vi "Test Remove Nested Test Class from Suite.vi"(8 "error in (no error)":errorcluster, 11 "LUnit Test Suite Tests in":refnum<class "LUnit Test Suite Tests.lvclass">) -> (0 "error out":errorcluster, 3 "LUnit Test Suite Tests out":refnum<class "LUnit Test Suite Tests.lvclass">)   [LabVIEW 2020, in "LUnit Test Suite Tests.lvclass"]
uses:
  LUnit Test Suite Tests.lvclass
  C:/Program Files (x86)/National Instruments/LabVIEW 2020/vi.lib/Astemes/LUnit/Test Case.lvclass
  Test Doubles/Test Case Test Double/Test Case Test Double.lvclass
  <vilib>/Astemes/LUnit/Test Case.lvclass/Test Case.ctl
  <vilib>/Astemes/LUnit/Core/LUnit Test Case/Private/Append Fail Result.vi
  <vilib>/Astemes/LUnit/Core/LUnit Test Case/Private/Append Pass Result.vi
  <vilib>/Astemes/LUnit/Core/LUnit Test Case/Private/Run In UI.vi
  <vilib>/Utility/error.llb/Clear Errors.vi
  source/Core/LUnit Test Suite/LUnit Test Suite.lvclass
  C:/git/astemes-lunit/source/Core/Runnable/Runnable.lvclass
  <vilib>/Astemes/LUnit/Test Case.lvclass
panel:
  out "List of Runnables":string[](array[string])
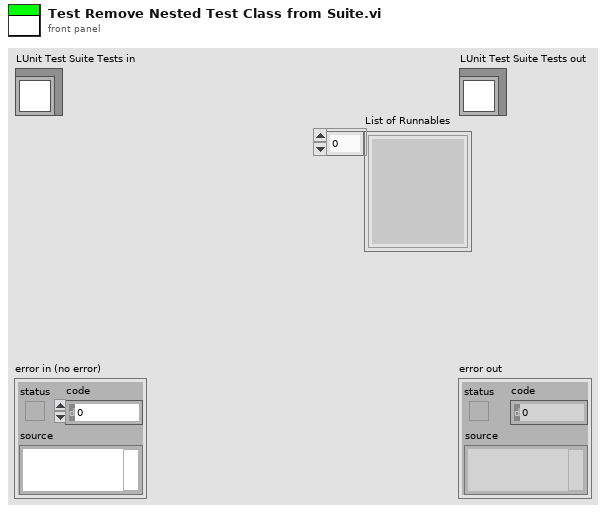
[diagram p1: front panel]
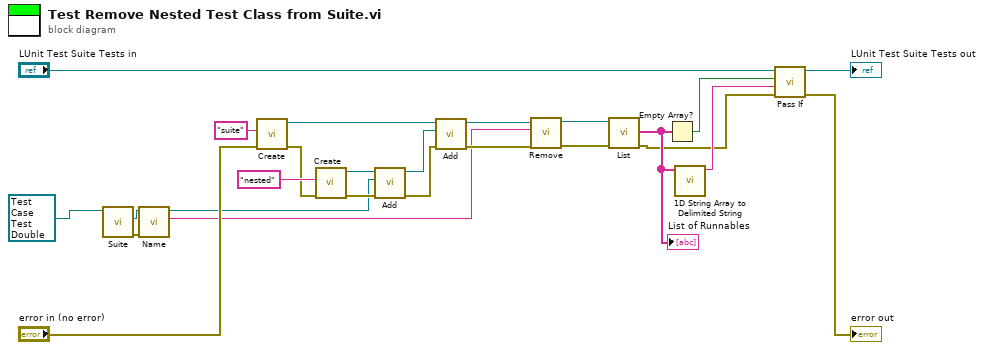
[diagram p0: block diagram]
diagram:
  n1 = call-dynamic "Suite.vi"("LUnit Test Case In"=refnum<class "Test Case Test Double.lvclass"> refnum ("Test Case Test Double.lvclass")) -> ("error out"=w10:errorcluster, "LUnit Test Suite Out"=w9:refnum<class "LUnit Test Suite.lvclass">)  [unwired: 8 in, 1 out]
  n2 = call-dynamic "Name.vi"("error in (no error)"=w10, "LUnit Test Suite in"=w9) -> ("Name"=w8:string, "LUnit Test Suite out"=w3:refnum<class "LUnit Test Suite.lvclass">)  [unwired: 7 in, 1 out]
  n3 = call "Create.vi"("error in (no error)"="error in (no error)", "Suite Name"="suite") -> ("error out"=w2:errorcluster, "LUnit Test Suite Out"=w24:refnum<class "LUnit Test Suite.lvclass">)  [unwired: 8 in]
  n4 = call "Create.vi"("error in (no error)"=w2, "Suite Name"="nested") -> ("error out"=w6:errorcluster, "LUnit Test Suite Out"=w5:refnum<class "LUnit Test Suite.lvclass">)  [unwired: 8 in]
  n5 = call "Add.vi"("error in (no error)"=w6, "Runnable"=w3, "LUnit Test Suite In"=w5) -> ("error out"=w1:errorcluster, "LUnit Test Suite Out"=w4:refnum<class "LUnit Test Suite.lvclass">)  [unwired: 7 in]
  n6 = call "Add.vi"("error in (no error)"=w1, "Runnable"=w4, "LUnit Test Suite In"=w24) -> ("error out"=w22:errorcluster, "LUnit Test Suite Out"=w23:refnum<class "LUnit Test Suite.lvclass">)  [unwired: 7 in]
  n7 = call "Remove.vi"("error in (no error)"=w22, "Test to Remove"=w8, "LUnit Test Suite In"=w23) -> ("error out"=w20:errorcluster, "LUnit Test Suite Out"=w21:refnum<class "LUnit Test Suite.lvclass">)  [unwired: 7 in]
  n8 = call "List.vi"("error in (no error)"=w20, "LUnit Test Suite In"=w21) -> ("error out"=w13:errorcluster, "List of Runnables"=w15:string[])  [unwired: 8 in]
  "List of Runnables" <- w15
  n9 = Empty Array?(array=w15) -> (empty?=w16:bool)
  n10 = call <vilib>:"1D String Array to Delimited String.vi"("string array"=w15) -> ("delimited string"=w14:string)  [unwired: 10 in]
  n11 = call <vilib>:"Pass If.vi"("error in (no error)"=w13, "Message"=w14, "Pass?"=w16, "LUnit Test Case In"="LUnit Test Suite Tests in") -> ("error out"=→"error out":errorcluster, "LUnit Test Case Out"=→"LUnit Test Suite Tests out":refnum<class "LUnit Test Suite Tests.lvclass">)  [unwired: 6 in]
